vi "SetData.vi"(0 "reference in":refnum<class "CustomersBase.lvclass">, 1 "Data":refnum<class "DataObject.lvclass">, 5 "error in (no error)":errorcluster) -> (14 "reference out":refnum<class "CustomersBase.lvclass">, 19 "error out":errorcluster)   [LabVIEW 2020, in "CustomersBase.lvclass"]
doc: "Property"
uses:
  CustomersBase.lvclass
  DataObject_class/DataObject.lvclass
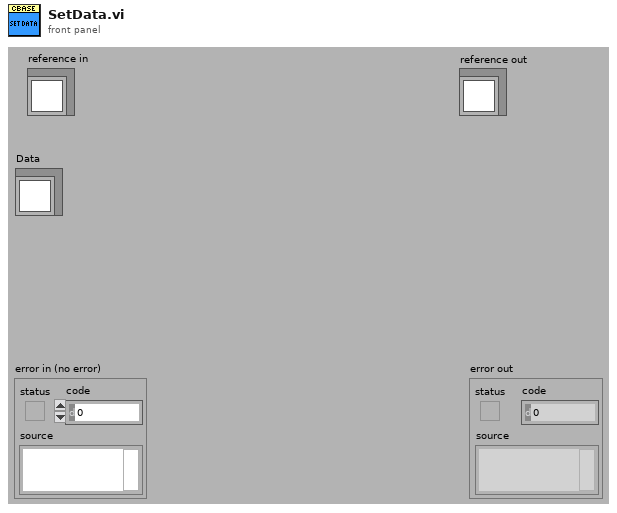
[diagram p1: front panel]
types:
  T1 = typedef "CustomersBase.lvclass/ObjectAttributes.ctl" = cluster{"_dataObject":refnum<class "DataObject.lvclass">, "Group":string}
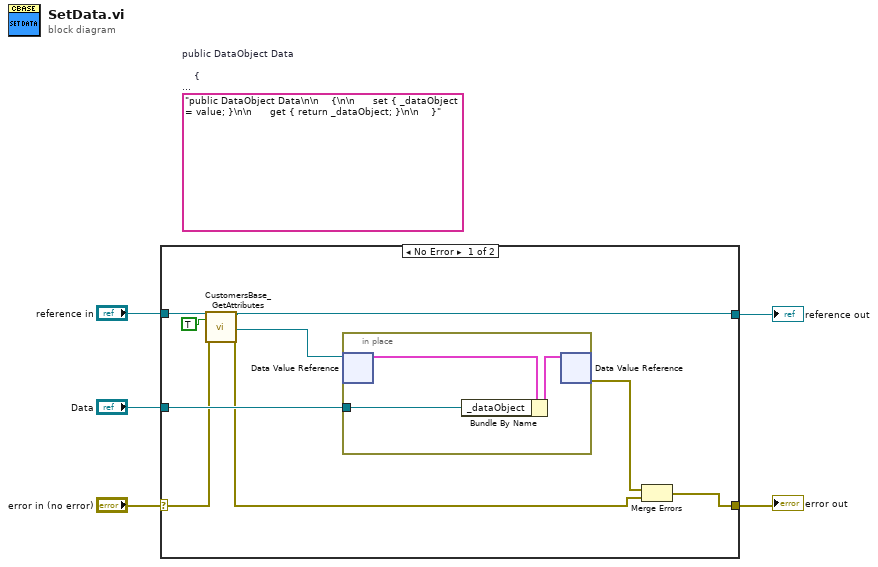
[diagram p0: block diagram]
diagram:
  (unwired) "public DataObject Data\n\n    {\n\n      set { _dataObject = value; }\n\n      get { return _dataObject; }\n\n    }"  # public DataObject Data      {        set { _dataObject = value; }        get { return _dataObject; }      }
  n1 = case shown="No Error" "error in (no error)" {
    selector: "error in (no error)" -> [w8 w19]
    tunnel: [w12 w19] -> w4
    tunnel: [w10 w18] -> w2
    tunnel: "reference in" -> [w11 w18]
    tunnel: "Data" -> [w14 _]
    frame No Error {
      n2 = call "CustomersBase_GetAttributes.vi"("reference in"=w11, "OnlyGetDvrReference(False)"=TRUE, "error in (no error)"=w8) -> ("reference out"=w10:refnum<class "CustomersBase.lvclass">, "DataRef"=w9:refnum<data-value>, "error out"=w7:errorcluster)  [unwired: 13 in, 1 out]
      n3 = in-place {
        in-place-border: w14 -> [w17]
        n4 = in-place-dvr #1(w9) -> (w16:T1)  [unwired: 1 out]
        n5 = Bundle By Name(cluster=w16, "_dataObject"=w17) -> (w15:T1)
        n6 = in-place-dvr #1(w15) -> (w13:errorcluster)  [unwired: 1 out]
      }
      n7 = Merge Errors(w13, w7) -> (w12:errorcluster)
    }
    frame Error {
    }
  }
  "error out" <- w4
  "reference out" <- w2
